vi "nirviSatArithMultEmu.vi"(2 "y":i16, 3 "x":i16) -> (0 "overflow":bool, 1 "x*y":i16)   [LabVIEW 2020]
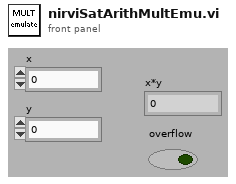
[diagram p1: front panel]
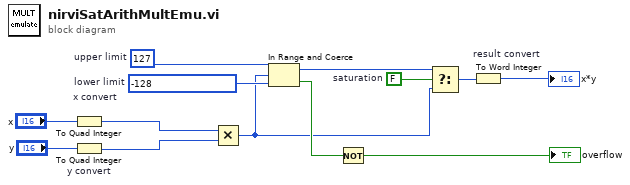
[diagram p0: block diagram]
diagram:
  w4 = i64 -128  # lower limit
  w5 = i64 127  # upper limit
  w9 = FALSE  # saturation
  n1 = To Quad Integer "x convert"(1:"x") -> (0:w3:i64)
  n2 = To Quad Integer "y convert"(1:"y") -> (0:w2:i64)
  n3 = Multiply(x=w3, y=w2) -> (x*y=w1:i64)
  n4 = In Range and Coerce(upper limit=w5, x=w1, lower limit=w4) -> (coerced(x)=w6:i64, In Range?=w7:bool)
  n5 = Not(x=w7) -> (.not. x?=→"overflow":bool)
  n6 = Select(t=w6, s=w9, f=w1) -> (s? t:f=w8:i64)
  n7 = To Word Integer "result convert"(number=w8) -> (16bit integer=→"x*y":i16)
